vi "Cube Vertices.vi"(4 "Scan Settings (um)":T1={"XStart"=1, "XEnd"=1, "XNum"=1, "YStart"=1, "YEnd"=1, "YNum"=1, "ZStart"=1, "ZEnd"=1, "ZNum"=1}, 6 "Scan Settings":T1={"XStart"=1, "XEnd"=1, "XNum"=1, "YStart"=1, "YEnd"=1, "YNum"=1, "ZStart"=1, "ZEnd"=1, "ZNum"=1}, 8 "error in":errorcluster, 9 "Points Selected":i32, 10 "In Points":i32[][](array[numeric]), 11 "AODAcq in":refnum<class "AODAcq.lvclass">) -> (0 "error out":errorcluster, 1 "Additional Points":i32, 2 "Out Points":i32[][](array[numeric]), 3 "AODAcq out":refnum<class "AODAcq.lvclass">)   [LabVIEW 2014, in "AODAcq.lvclass"]
uses:
  AODAcq.lvclass
panel:
  in  "Side Size um":dbl=2.0
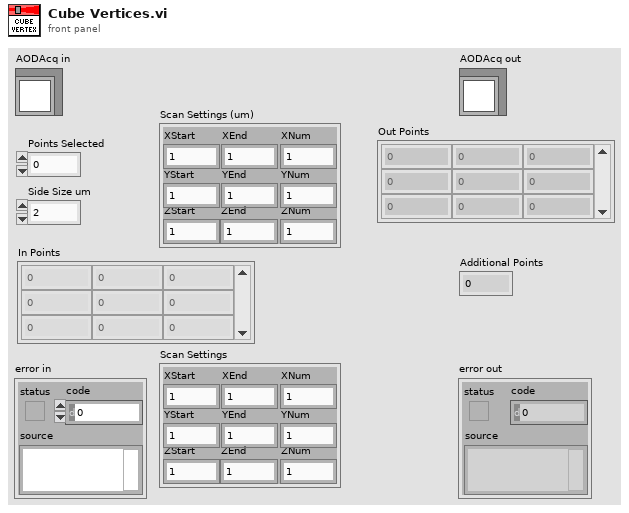
[diagram p1: front panel]
types:
  T1 = cluster{"XStart":i32, "XEnd":i32, "XNum":i32, "YStart":i32, "YEnd":i32, "YNum":i32, "ZStart":i32, "ZEnd":i32, "ZNum":i32}
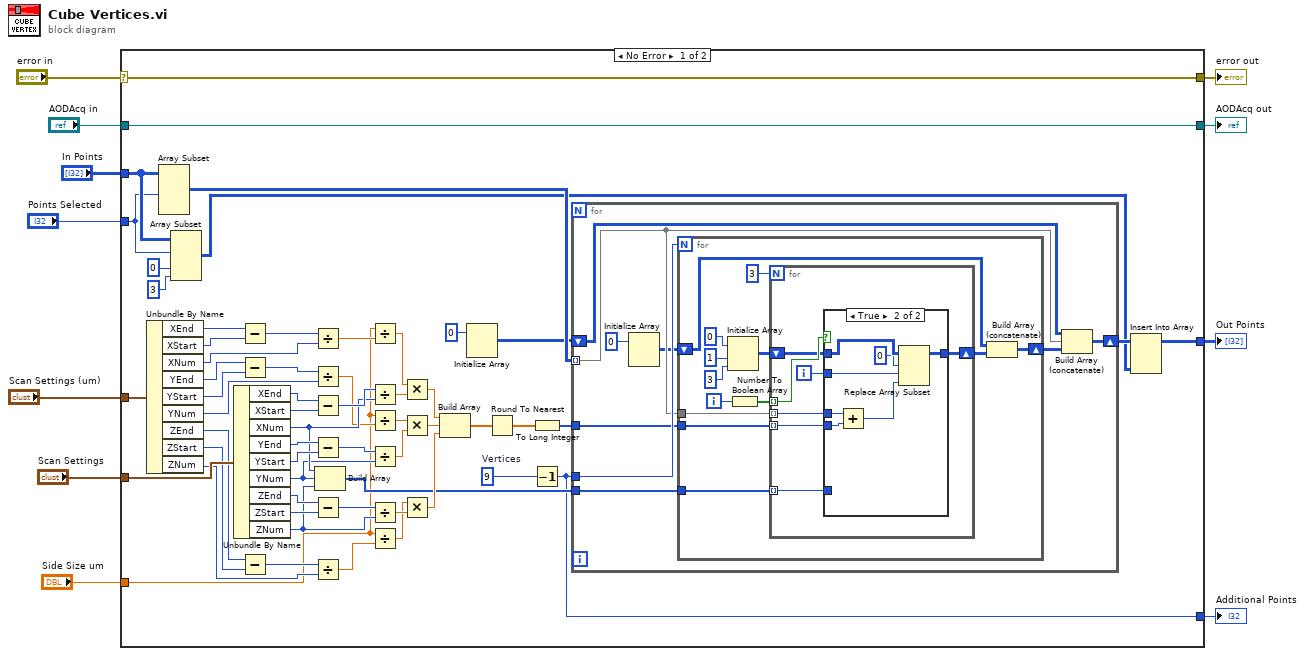
[diagram p0: block diagram]
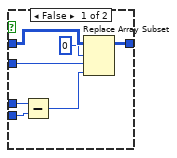
[diagram p2: hidden frame]
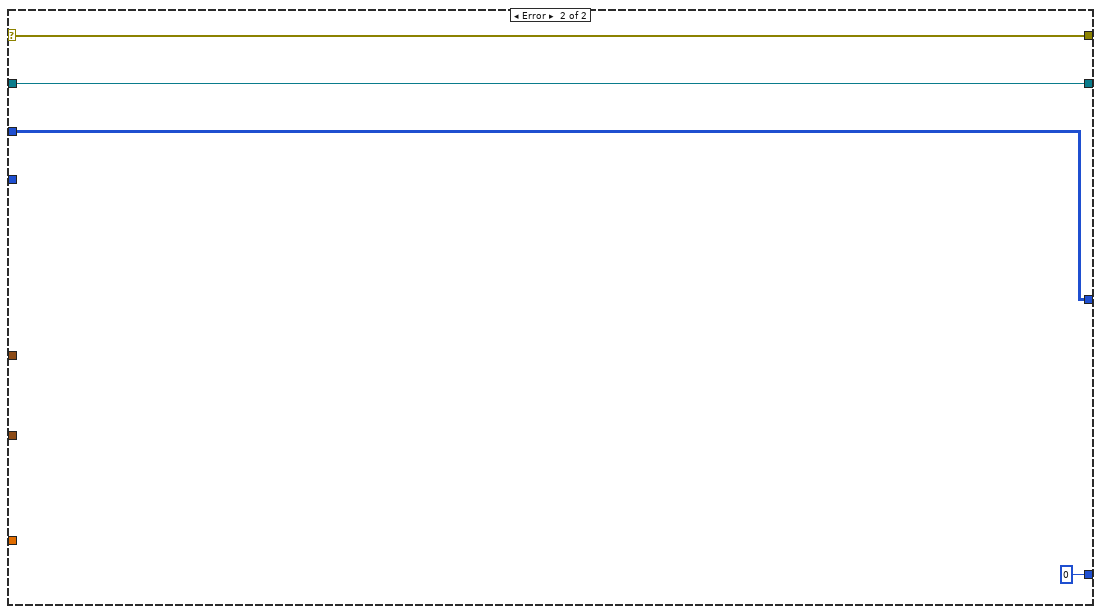
[diagram p3: hidden frame]
diagram:
  n1 = case shown="No Error" "error in" {
    selector: "error in" -> [w67 w115]
    tunnel: [w67 w115] -> w10
    tunnel: [w68 w114] -> w8
    tunnel: "AODAcq in" -> [w68 w114]
    tunnel: "Scan Settings" -> [w66 _]
    tunnel: "Side Size um" -> [w27 _]
    tunnel: "In Points" -> [w21 w113]
    tunnel: "Points Selected" -> [w20 _]
    tunnel: "Scan Settings (um)" -> [w42 _]
    tunnel: [w15 w113] -> w2
    tunnel: [w14 0] -> w1
    frame No Error {
      w43 = 9  # Vertices
      n2 = Unbundle By Name(w42) -> ("XEnd"=w41:i32, "XStart"=w40:i32, "XNum"=w34:i32, "YEnd"=w39:i32, "YStart"=w36:i32, "YNum"=w32:i32, "ZEnd"=w38:i32, "ZStart"=w37:i32, "ZNum"=w30:i32)
      n3 = Array Subset(array=w21, length (row)=w20) -> (w49:i32[][])  [unwired: 3 in]
      n4 = Array Subset(array=w21, index (row)=w20, index (col)=0 ("index"), length (col)=3 ("length")) -> (w16:i32[][])  [unwired: 1 in]
      n5 = Unbundle By Name(w66) -> ("XEnd"=w64:i32, "XStart"=w65:i32, "XNum"=w47:i32, "YEnd"=w63:i32, "YStart"=w62:i32, "YNum"=w46:i32, "ZEnd"=w61:i32, "ZStart"=w60:i32, "ZNum"=w45:i32)
      n6 = Subtract(x=w41, y=w40) -> (x-y=w35:i32)
      n7 = Subtract(x=w39, y=w36) -> (x-y=w33:i32)
      n8 = Subtract(x=w38, y=w37) -> (x-y=w31:i32)
      n9 = Divide(x=w35, y=w34) -> (x/y=w29:dbl)
      n10 = Divide(x=w33, y=w32) -> (x/y=w28:dbl)
      n11 = Subtract(x=w64, y=w65) -> (x-y=w59:i32)
      n12 = Subtract(x=w63, y=w62) -> (x-y=w58:i32)
      n13 = Subtract(x=w61, y=w60) -> (x-y=w57:i32)
      n14 = Divide(x=w31, y=w30) -> (x/y=w26:dbl)
      n15 = Build Array(w47, w46, w45) -> (w44:i32[])
      n16 = Divide(x=w27, y=w29) -> (x/y=w25:dbl)
      n17 = Divide(x=w59, y=w47) -> (x/y=w56:dbl)
      n18 = Divide(x=w27, y=w28) -> (x/y=w24:dbl)
      n19 = Divide(x=w58, y=w46) -> (x/y=w55:dbl)
      n20 = Divide(x=w57, y=w45) -> (x/y=w54:dbl)
      n21 = Divide(x=w27, y=w26) -> (x/y=w23:dbl)
      n22 = Multiply(x=w25, y=w56) -> (x*y=w53:dbl)
      n23 = Multiply(x=w24, y=w55) -> (x*y=w52:dbl)
      n24 = Multiply(x=w23, y=w54) -> (x*y=w51:dbl)
      n25 = Build Array(w53, w52, w51) -> (w22:dbl[])
      n26 = Initialize Array(0 ("element")) -> (w12:i32[][])  [unwired: 2 in]
      n27 = Round To Nearest(number=w22) -> (nearest integer value=w50:dbl[])
      n28 = To Long Integer(number=w50) -> (32bit integer=w48:i32[])
      n29 = Decrement(x=w43) -> (x-1=w14:i32)
      n30 = for {
        tunnel: w49 -> [w75] mode=indexing
        shift-right: [w71] -> w17
        shift-left: w12 -> [w77]
        tunnel: w14 -> [w76]
        tunnel: w48 -> [w69]
        tunnel: w44 -> [w72]
        n31 = Initialize Array(0 ("element")) -> (w73:i32[][])  [unwired: 2 in]
        n32 = for {
          N: w76 -> [_]
          tunnel: w69 -> [w84]
          tunnel: w75 -> [w83]
          shift-right: [w79] -> w70
          shift-left: w73 -> [w82]
          tunnel: w72 -> [w80]
          i -> [w90]
          n33 = Initialize Array(0 ("element"), 1 ("dimension size"), 3 ("dimension size")) -> (w86:i32[][])
          n34 = Number To Boolean Array(number=w90) -> (Boolean array=w88:bool[])
          n35 = for {
            N: 3 -> [_]
            tunnel: w88 -> [w97] mode=indexing
            shift-right: [w92] -> w81
            shift-left: w86 -> [w96]
            tunnel: w84 -> [w94] mode=indexing
            tunnel: w83 -> [w93] mode=indexing
            tunnel: w80 -> [w91] mode=indexing
            i -> [w95]
            n36 = case shown="True" w97 {
              tunnel: w96 -> [w104 w111]
              tunnel: w95 -> [w100 w106]
              tunnel: w94 -> [w102 w109]
              tunnel: w93 -> [w103 w110]
              tunnel: [w101 w108] -> w92
              tunnel: w91 -> [_ _]
              frame False {
                n37 = Subtract(x=w103, y=w102) -> (x-y=w98:i32)
                n38 = Replace Array Subset(array=w104, new element=w98, index (row)=0 ("disabled index (row)"), index (col)=w100) -> (w101:i32[][])
              }
              frame True {
                n39 = Add(x=w110, y=w109) -> (x+y=w105:i32)
                n40 = Replace Array Subset(array=w111, new element=w105, index (row)=0, index (col)=w106) -> (w108:i32[][])
              }
            }
          }
          n41 = Build Array (concatenate)(w82, w81) -> (w79:i32[][])
        }
        n42 = Build Array (concatenate)(w77, w75, w70) -> (w71:i32[][])
      }
      n43 = Insert Into Array(array=w17, new element=w16) -> (w15:i32[][])  [unwired: 2 in]
    }
    frame Error {
    }
  }
  "error out" <- w10
  "AODAcq out" <- w8
  "Out Points" <- w2
  "Additional Points" <- w1
